vi "Actor Core.vi"(8 "error in":errorcluster, 11 "RDS Helm Actor in":refnum<class "RDS Helm Actor.lvclass">) -> (0 "error out":errorcluster, 3 "Actor out":refnum<class "Actor.lvclass">)   [LabVIEW 2015, in "RDS Helm Actor.lvlib" / "RDS Helm Actor.lvclass"]
doc: "(<B>Filename</B>: Actor Framework.lvlib:Actor.lvclass:Actor Core.vi)\n\nReceives messages to the actor, reacts to them, and initiates any error handling that may shut the actor down.\n\nDescendant classes may override this VI to append parallel tasks for the actor to complete while it handles messages. Overrides use the Call Parent Method node."
uses:
  RDS Helm Actor.lvclass
  <vilib>/ActorFramework/Actor/Actor.lvclass
  RDS Helm Actor.lvclass/RDS Helm Actor.ctl
  <vilib>/ActorFramework/Actor/Actor.lvclass/Actor.ctl
  <vilib>/ActorFramework/Message Enqueuer/Message Enqueuer.lvclass/Message Enqueuer.ctl
  <vilib>/ActorFramework/Message Enqueuer/Init from Existing Queue.vi
  <vilib>/ActorFramework/Message Enqueuer/Message Enqueuer.lvclass
  RDS Parent Actor/RDS Parent Actor/RDS Parent Actor.lvclass
  RDS Helm Actor Messages/Helm State Machine Cycle Msg/Helm State Machine Cycle Msg.lvclass
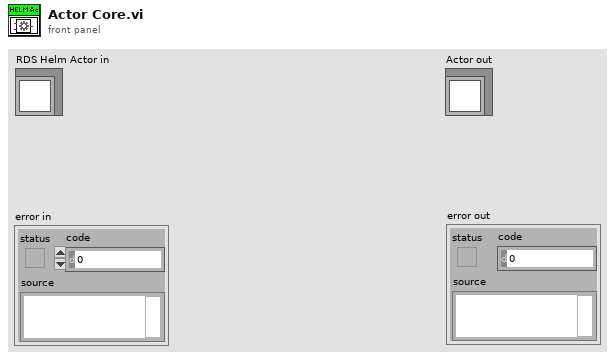
[diagram p1: front panel]
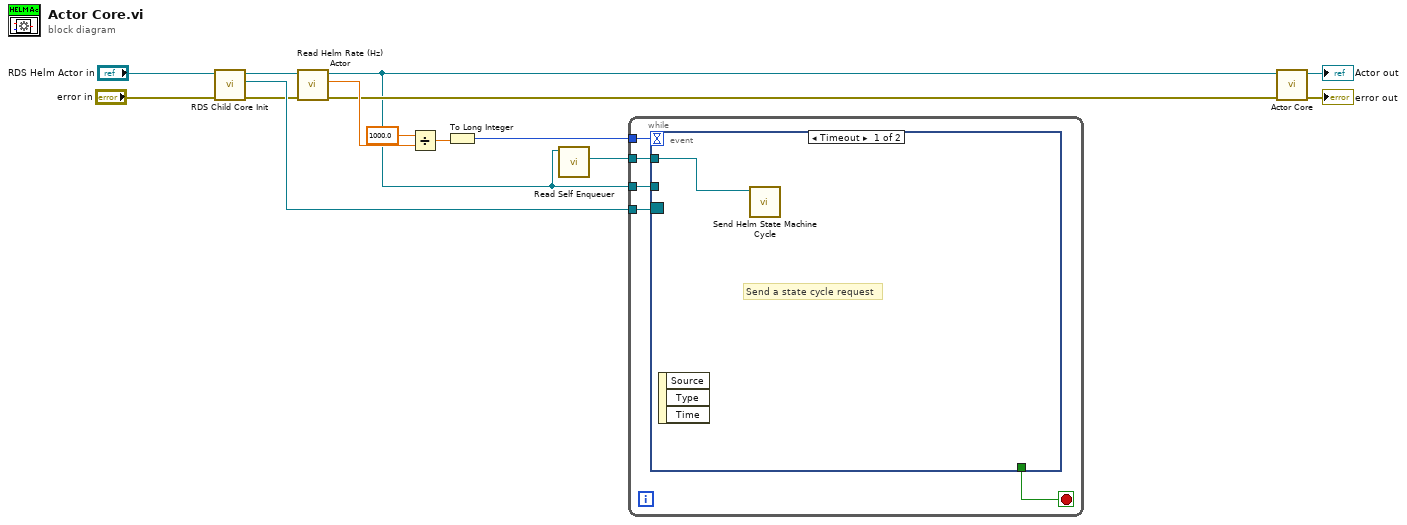
[diagram p0: block diagram]
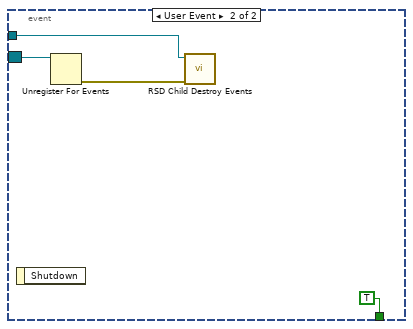
[diagram p2: hidden frame]
diagram:
  n1 = call "RDS Child Core Init.vi"("error in (no error)"="error in", "RDS Parent Actor in"="RDS Helm Actor in") -> ("error out"=w6:errorcluster, "Event Registration Refnum"=w10:refnum<event-registration>, "RDS Parent Actor out"=w7:refnum<class "RDS Helm Actor.lvclass">)  [unwired: 6 in, 1 out]
  n2 = call "Read Helm Rate (Hz) Actor.vi"("error in (no error)"=w6, "RDS Helm Actor in"=w7) -> ("error out"=w4:errorcluster, "Helm Rate (Hz)"=w5:dbl, "RDS Helm Actor out"=w3:refnum<class "RDS Helm Actor.lvclass">)  [unwired: 7 in]
  n3 = Divide(x=1000.0, y=w5) -> (x/y=w11:dbl)
  n4 = To Long Integer(number=w11) -> (32bit integer=w1:i32)
  n5 = call <vilib>:"Read Self Enqueuer.vi"("Actor"=w3) -> ("Self Enqueuer"=w2:refnum<class "Message Enqueuer.lvclass">)  [unwired: 10 in]
  n6 = while {
    tunnel: w10 -> [w18]
    tunnel: w3 -> [w19]
    tunnel: w1 -> [w16]
    tunnel: w2 -> [w15]
    stop <- w17 stop-if-true
    n7 = event shown="[0] Timeout" {
      selector: w18 -> [_ w22]
      dyn-events: _ -> [_ _]
      timeout: w16 -> [_ _]
      tunnel: w19 -> [_ w21]
      tunnel: [_ TRUE] -> w17
      tunnel: w15 -> [w20 _]
      event Timeout {
        # "Send a state cycle request"
        n8 = event-data() -> ()  [unwired: 1 in, 3 out]
        n9 = call "Send Helm State Machine Cycle.vi"("Message Enqueuer in"=w20) -> ()  [unwired: 9 in, 2 out]
      }
      event User Event {
        n10 = event-data() -> ()  [unwired: 1 in, 1 out]
        n11 = Unregister For Events(event registration refnum=w22) -> (error out=w23:errorcluster)  [unwired: 1 in]
        n12 = call "RSD Child Destroy Events.vi"("error in (no error)"=w23, "RDS Parent Actor in"=w21) -> ()  [unwired: 8 in, 2 out]
      }
    }
  }
  n13 = call-parent "Actor Core.vi"("error in"=w4, "Actor in"=w3) -> ("error out"=→"error out":errorcluster, "Actor out"=→"Actor out":refnum<class "Actor.lvclass">)  [unwired: 8 in]
